vi "Log Event.vi"(0 "Robot Notifications in":refnum<class "Robot Event.lvclass">, 1 "Program":string, 2 "data":variant, 5 "error in (no error)":errorcluster, 9 "Event Type":T1) -> (14 "Robot Notifications out":refnum<class "Robot Event.lvclass">, 19 "error out":errorcluster)   [LabVIEW 2019, in "Robot Event.lvclass"]
uses:
  Robot Event.lvclass
  Event Type.ctl
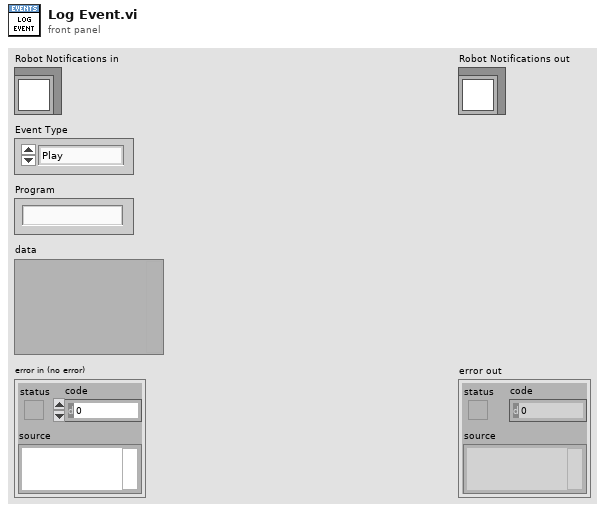
[diagram p1: front panel]
types:
  T1 = typedef "Robot Event.lvclass/Event Type.ctl" = enum16{"Play", "Error", "Fault", "Timeout", "Fault - Program Resumed", "Fault - Program Aborted"}
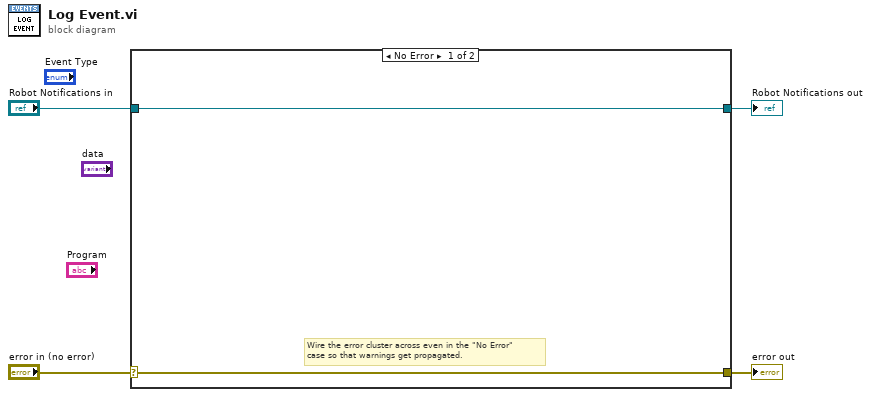
[diagram p0: block diagram]
diagram:
  n1 = case shown="No Error" "error in (no error)" {
    selector: "error in (no error)" -> [w5 w8]
    tunnel: [w5 w8] -> w3
    tunnel: [w6 w7] -> w1
    tunnel: "Robot Notifications in" -> [w6 w7]
    frame No Error {
      # "Wire the error cluster across even in the \"No Error\"\ncase so that warnings get propagated."
    }
    frame Error {
    }
  }
  "error out" <- w3
  "Robot Notifications out" <- w1
